vi "Reset Run Count.vi"(8 "error in (no error)":errorcluster, 11 "CommandDirector in":refnum<class "CommandDirector.lvclass">) -> (0 "error out":errorcluster, 3 "CommandDirector out":refnum<class "CommandDirector.lvclass">)   [LabVIEW 2023, in "HAF.lvlib" / "CommandDirector.lvclass"]
doc: "Resets the Run Count to zero."
uses:
  CommandDirector.lvclass
  CommandDirector.lvclass/CommandDirector.ctl
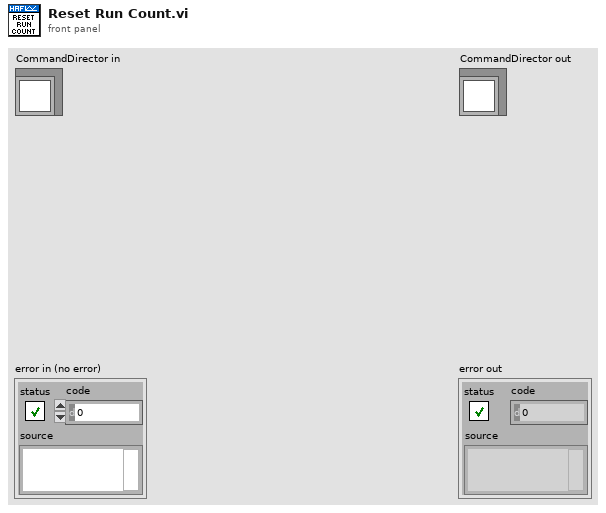
[diagram p1: front panel]
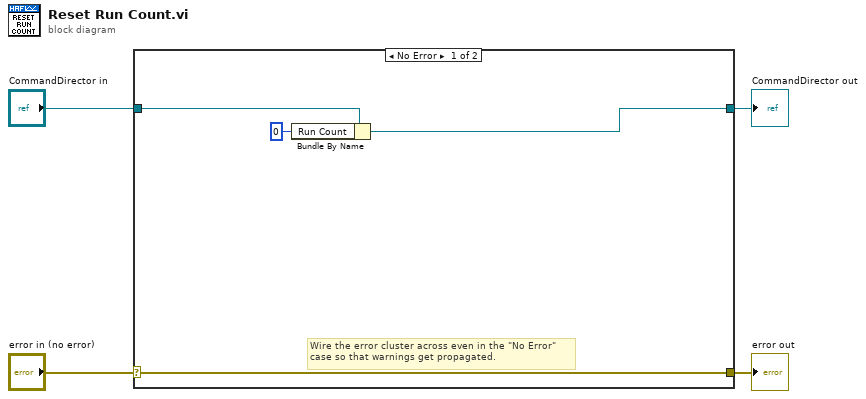
[diagram p0: block diagram]
diagram:
  n1 = case shown="No Error" "error in (no error)" {
    selector: "error in (no error)" -> [w8 w10]
    tunnel: [w8 w10] -> w3
    tunnel: [w6 w9] -> w1
    tunnel: "CommandDirector in" -> [w7 w9]
    frame No Error {
      # "Wire the error cluster across even in the \"No Error\"\ncase so that warnings get propagated."
      n2 = Bundle By Name(cluster=w7, "Run Count"=u32 0) -> (w6:refnum<class "CommandDirector.lvclass">)
    }
    frame Error {
    }
  }
  "error out" <- w3
  "CommandDirector out" <- w1
